vi "countdown-timer.vi"(6 "Timer-c in":dbl, 7 "switches":bool, 9 "Timer-s in":dbl, 10 "Timer C Ref":refnum<vi>, 11 "Timer S Ref":refnum<vi>) -> (1 "Stop Timer":bool, 2 "Timer-c out":dbl, 3 "Timer-s out":dbl)   [LabVIEW 2021]
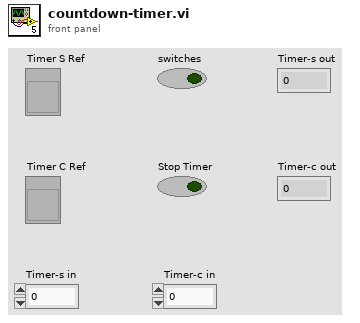
[diagram p1: front panel]
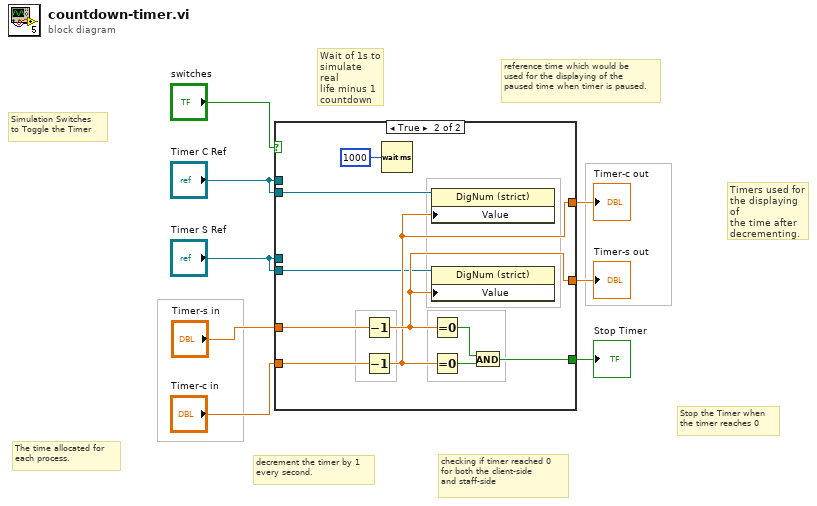
[diagram p0: block diagram]
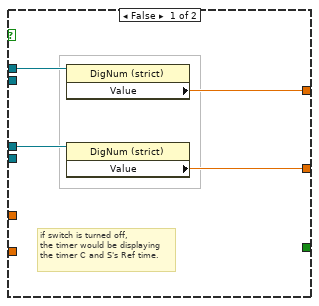
[diagram p2: hidden frame]
diagram:
  # "Timers used for\nthe displaying of\nthe time after\ndecrementing."
  # "The time allocated for\neach process."
  # "reference time which would be\nused for the displaying of the\npaused time when timer is paused."
  # "Wait of 1s to\nsimulate real\nlife minus 1\ncountdown"
  # "Simulation Switches\nto Toggle the Timer"
  # "Stop the Timer when\nthe timer reaches 0"
  # "checking if timer reached 0\nfor both the client-side\nand staff-side"
  # "decrement the timer by 1\nevery second."
  n1 = case shown="True" "switches" {
    tunnel: [_ w18] -> w3
    tunnel: "Timer-s in" -> [_ w22]
    tunnel: "Timer-c in" -> [_ w21]
    tunnel: [w12 w17] -> w6
    tunnel: [w11 w16] -> w7
    tunnel: "Timer S Ref" -> [w10 _]
    tunnel: "Timer C Ref" -> [w9 _]
    tunnel: "Timer S Ref" -> [_ w14]
    tunnel: "Timer C Ref" -> [_ w13]
    frame False {
      # "if switch is turned off,\nthe timer would be displaying\nthe timer C and S's Ref time."
      n2 = property class="DigNum (strict)"(reference=w9) -> ("Value"=w11:dbl)  [unwired: 1 in, 2 out]
      n3 = property class="DigNum (strict)"(reference=w10) -> ("Value"=w12:dbl)  [unwired: 1 in, 2 out]
    }
    frame True {
      n4 = Decrement(x=w22) -> (x-1=w17:dbl)
      n5 = Decrement(x=w21) -> (x-1=w16:dbl)
      n6 = Wait (ms)(milliseconds to wait=u32 1000) -> ()  [unwired: 1 out]
      n7 = property class="DigNum (strict)"(reference=w13, "Value"=w16) -> ()  [unwired: 1 in, 2 out]
      n8 = property class="DigNum (strict)"(reference=w14, "Value"=w17) -> ()  [unwired: 1 in, 2 out]
      n9 = Equal To 0?(x=w17) -> (x = 0?=w20:bool)
      n10 = Equal To 0?(x=w16) -> (x = 0?=w19:bool)
      n11 = And(x=w20, y=w19) -> (x .and. y?=w18:bool)
    }
  }
  "Timer-c out" <- w7
  "Timer-s out" <- w6
  "Stop Timer" <- w3
